vi "write commands.vi"(0 "Video to Inject":path=path "C:/ProgramData/LabVIEWEval/Protected/19 - Block Diagram Demonstration Summary.mp4", 7 "Commands":cluster{"output 7":dbl, "Instruction":string}[](array[cluster])=[{"output 7"=18.780358, "Instruction"="open main.vi"}, {"output 7"=25.204399, "Instruction"="open block diagram"}, {"output 7"=45.571315, "Instruction"="push hot-key to show menu bar"}, {"output 7"=67.59345, "Instruction"="objhiglight terminals"}, {"output 7"=82.594252, "Instruction"="show frontpanel terminals to one"}, {"output 7"=100.064171, "Instruction"="show different terminal types"}, {"output 7"=156.39976, "Instruction"="highlight express VI"}, {"output 7"=171.581377, "Instruction"="highlight mic input"}, {"output 7"=177.513166, "Instruction"="highlight spectral"}, {"output 7"=191.033137, "Instruction"="highlight wire connecting the two"}, {"output 7"=216.004836, "Instruction"="highlight chart"}, {"output 7"=223.317873, "Instruction"="highlight while loop"}, {"output 7"=236.029946, "Instruction"="highlight run VI button and run"}], 11 "error in":errorcluster) -> (15 "error out":errorcluster)   [LabVIEW 2026]
uses:
  7bea4fd5-ddf4-473e-a7a1-0f8fbfc0b8ea.vi
  9cb9b53c-b5ec-4711-9642-681976bee622.vi
  <vilib>/JDP Science/JSONtext/JSON text to Variant.vi
  <vilib>/JDP Science/JSONtext/Variant to JSON Text.vi
  <vilib>/JDP Science/JSONtext/LVClass Serializer/JSONtext LVClass Serializer.lvclass
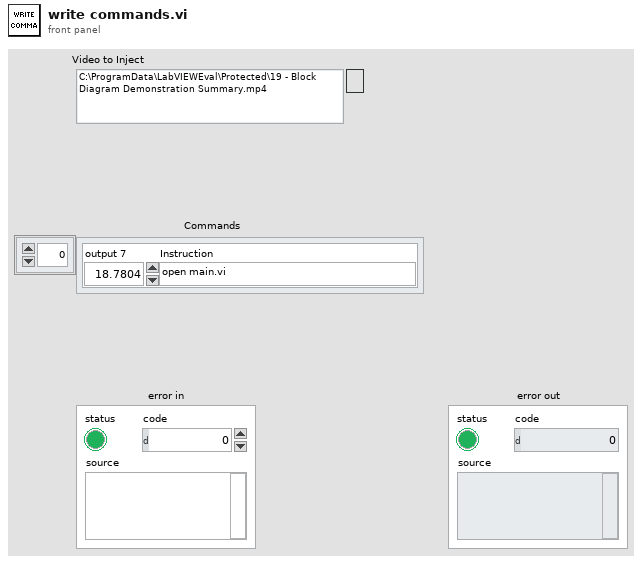
[diagram p1: front panel]
types:
  T1 = enum16{"open", "replace", "create", "open or create", "replace or create", "replace or create with confirmation"}
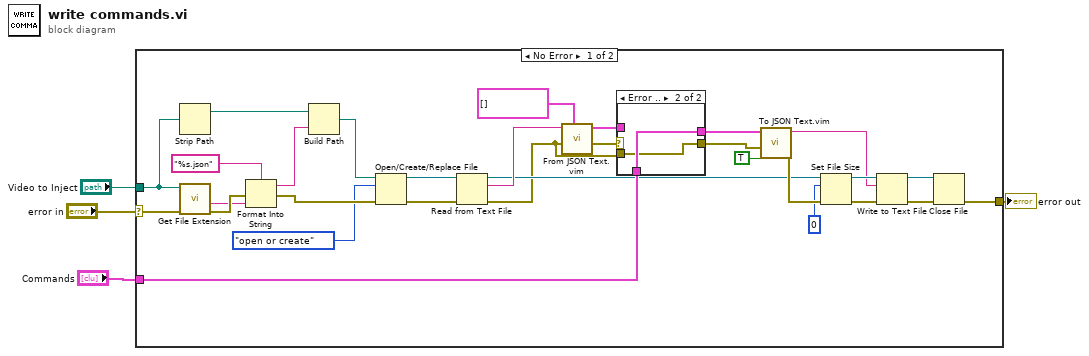
[diagram p0: block diagram]
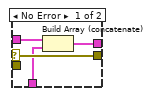
[diagram p2: hidden frame]
diagram:
  n1 = case shown="No Error" "error in" {
    selector: "error in" -> [w29 w41]
    tunnel: "Video to Inject" -> [w24 _]
    tunnel: "Commands" -> [w13 _]
    tunnel: [w25 w41] -> w3
    frame No Error {
      n2 = Strip Path(path=w24) -> (stripped path=w21:path)  [unwired: 1 out]
      n3 = call <vilib>:"Get File Extension.vi"("error in (no error)"=w29, "file"=w24) -> ("error out"=w28:errorcluster, "filename without extension"=w23:string)  [unwired: 5 in, 3 out]
      n4 = Format Into String(format string="%s.json", error in=w28, w23) -> (resulting string=w20:string, error out=w27:errorcluster)  [unwired: 1 in]
      n5 = Build Path(base path=w21, name or relative path=w20) -> (appended path=w18:path)
      n6 = Open/Create/Replace File(file path (use dialog)=w18, error in=w27, operation (0:open)=T1."open or create") -> (refnum out=w16:refnum<file>, error out=w33:errorcluster)  [unwired: 3 in, 1 out]
      n7 = Read from Text File(file (use dialog)=w16, error in=w33) -> (refnum out=w10:refnum<file>, text=w15:string, error out=w5:errorcluster)  [unwired: 2 in, 1 out]
      n8 = call "From JSON Text.vim"("Data Type and Default Value"=cluster{"output 7":dbl, "Instruction":string}[] [] ("appended array"), "error in (no error)"=w5, "JSON"=w15) -> ("error out"=w32:errorcluster, "Data out"=w14:cluster{"output 7":dbl, "Instruction":string}[])  [unwired: 7 in]
      n9 = case shown="Error .." w32 {
        selector: w32 -> [w38 _]
        tunnel: w14 -> [w37 _]
        tunnel: [w36 w40] -> w11
        tunnel: w13 -> [w35 w40]
        tunnel: [w38 w39] -> w26
        tunnel: w5 -> [_ w39]
        frame No Error {
          n10 = Build Array (concatenate)(w37, w35) -> (w36:cluster{"output 7":dbl, "Instruction":string}[])
        }
        frame Error {
        }
      }
      n11 = call "To JSON Text.vim"("Pretty Print?"=TRUE, "error in (no error)"=w26, "Anything"=w11) -> ("error out"=w30:errorcluster, "<JSON>"=w7:string)  [unwired: 7 in]
      n12 = Set File Size(4:w30, 6:i64 0 ("size (in bytes)"), 7:w10) -> (0:w31:errorcluster, 3:w9:refnum<file>)
      n13 = Write to Text File(file (use dialog)=w9, text=w7, error in=w31) -> (refnum out=w8:refnum<file>, error out=w34:errorcluster)  [unwired: 1 in, 1 out]
      n14 = Close File(refnum=w8, error in=w34) -> (error out=w25:errorcluster)  [unwired: 1 out]
    }
    frame Error {
    }
  }
  "error out" <- w3
